vi "RequiredForAll-Mode.vi"(8 "error in (no error)":errorcluster, 11 "CAN-NI in":refnum<class "CAN-NI.lvclass">) -> (0 "error out":errorcluster, 2 "Mode":T1=enum."LabVIEW(DriverLayer)", 3 "CAN-NI out":refnum<class "CAN-NI.lvclass">)   [LabVIEW 2019, in "CAN-NI.lvlib" / "CAN-NI.lvclass"]
uses:
  CAN-NI.lvclass
  <vilib>/lvAPT/.lib/HAL-Interface.lvlibp/HALInterface/Typedef/Def-Mode.ctl
  <vilib>/lvAPT/.lib/HAL-Interface.lvlibp/HALInterface/HALInterface.lvclass
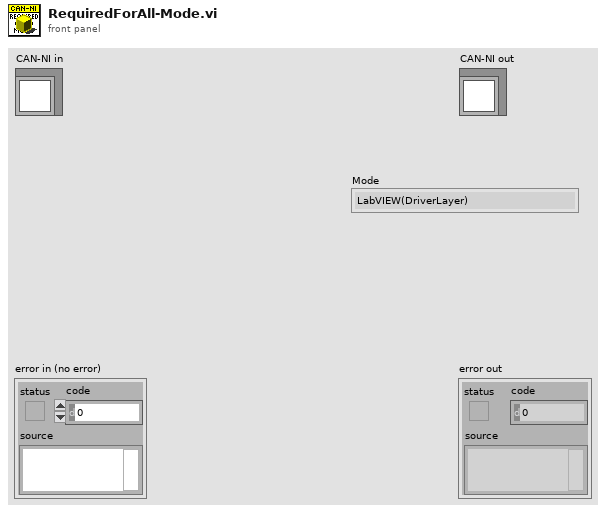
[diagram p1: front panel]
types:
  T1 = typedef "HAL-Interface.lvlibp/HALInterface.lvclass/Def-Mode.ctl" = enum16{"AbstractLayer", "LabVIEW(DriverLayer)", "DLL(DriverLayer)", "RPC(DriverLayer)"}
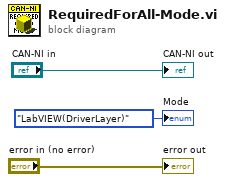
[diagram p0: block diagram]
diagram:
  "error out" <- "error in (no error)"
  "CAN-NI out" <- "CAN-NI in"
  "Mode" <- Def-Mode."LabVIEW(DriverLayer)" ("Mode")
